vi "I2C Utility Example EEPROM Write-and-Read.vi"() -> ()   [LabVIEW 2020]
panel:
  out "I2C_READ_DATA (Read)":u8[](array[numeric]) format="%x"
  out "Acks Received (Read)":dbl
  in  "I2C_NUM_BYTES_RX (Read)":i32=15
  in  "I2C_WRITE_DATA (Read)":i32[](array[numeric])=[0]
  out "I2C COM Error Out":errorcluster={"status"=FALSE, "code"=0, "source"="No Error"}
  in  "I2C_NUM_BYTES_RX (Write)":i32
  in  "I2C_WRITE_DATA (Write)":u8[](array[numeric])=[0, 222, 173, 190, 239, 1, 2, 3, 4, 5, 6, 7, 222, 173, 190, 239] format="%x"
  out "I2C_READ_DATA (Write)":u8[](array[numeric]) format="%x"
  out "Acks Received (Write)":dbl
  in  "I2C_SLAVE_ADDRESS":i32=80
  in  "I2C_OPTIONS":i32
  in  "I2C_SPEED_THROTTLE":i32
  in  "I2C_SCL_DIONUM":i32=1
  in  "I2C_SDA_DIONUM":i32
  out "Error String":string="No Error"
  out "error out":errorcluster
  out "ConnectionType Out":i32
  out "DeviceType Out":i32
  in  "Identifier":string="LJM_idANY"
  in  "ConnectionType":string="LJM_ctANY"
  in  "DeviceType":string="LJM_dtANY"
  # "Before running this program:\n1. Attach a LJTick-DAC to FIO0 and FIO1\n2. Configure Device Opening Settings (DeviceType, ConnectionType, and Identifier)\n3. Configure I2C Settings (I2C_SDA_DIONUM, I2C_SCL_DIONUM, I2C_SPEED_THROTTLE, I2C_OPTIONS, I2C_SLAVE_ADDRESS)\n4. Run the .vi by either 'ctrl+r' or by pressing the \"Run\" button.\n\nThis program combines the two VI's:\n\"I2C Utility Example EEPROM Write.vi\"\n\"I2C Utility Example EEPROM Read.vi\""
  # "Device Opening Settings"
  # "Data [0]"
  # "PageNum"
  # "Data [0]"
  # "PageNum"
  # "Data [0]"
  # "Data [1]"
  # "Data [1]"
  # "Data [2]"
  # "Data [2]"
  # "Data [1]"
  # "Data [3]"
  # "Data [2]"
  # "Data [3]"
  # "..."
  # "Data [3]"
  # "..."
  # "..."
  # "I2C Settings"
  # "Configures the FIO channel that the \nSDA signal should appear on."
  # "Configures the FIO channel that the \nSDA signal should appear on."
  # "Configures the I2C Clock Speed\n (frequency)"
  # "Configures the I2C options"
  # "..."
  # "..."
  # "Data [14]"
  # "Data [14]"
  # "..."
  # "Configure the slave address to be sent \nat the start of each data transfer"
  # "Data [14]"
  # "Errors:"
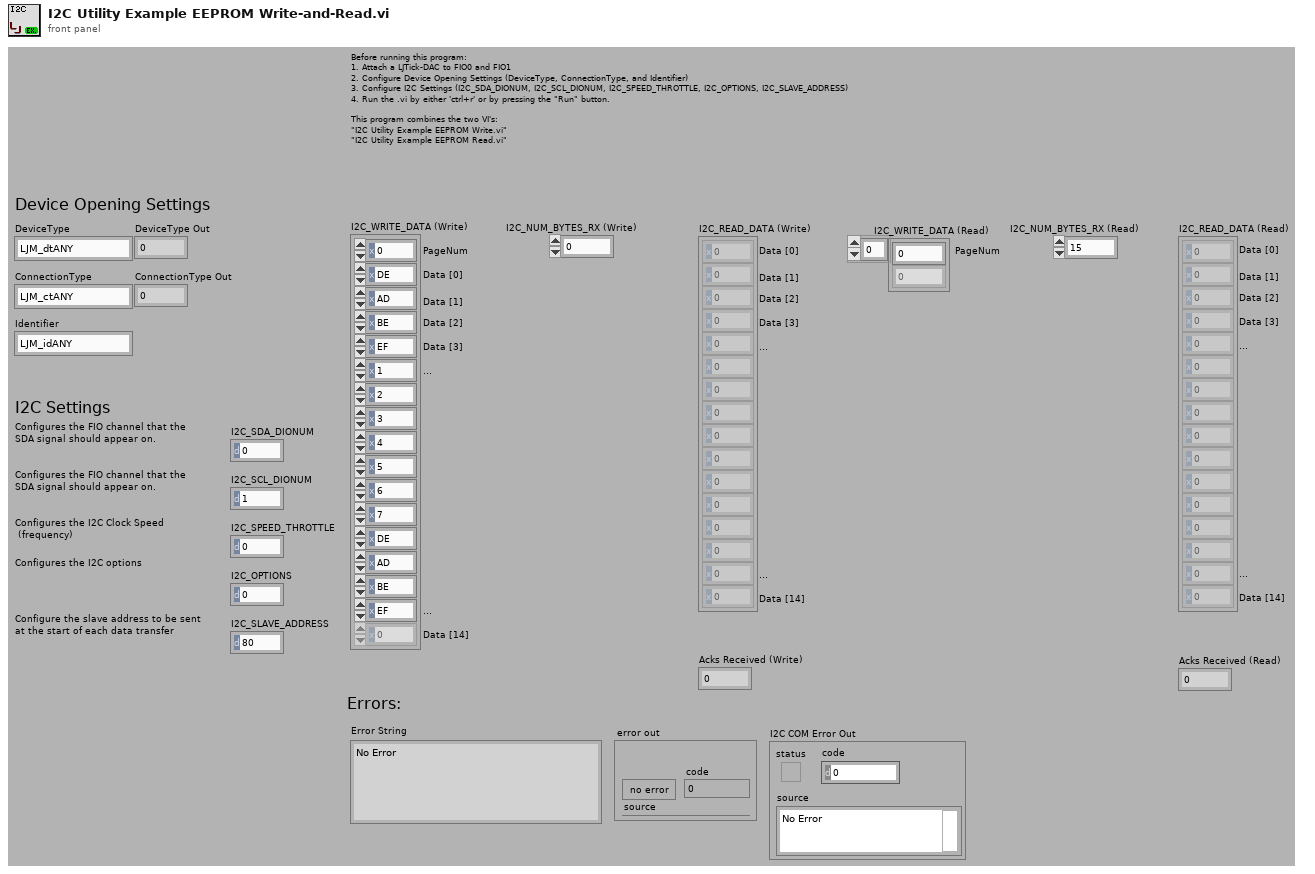
[diagram p1: front panel]
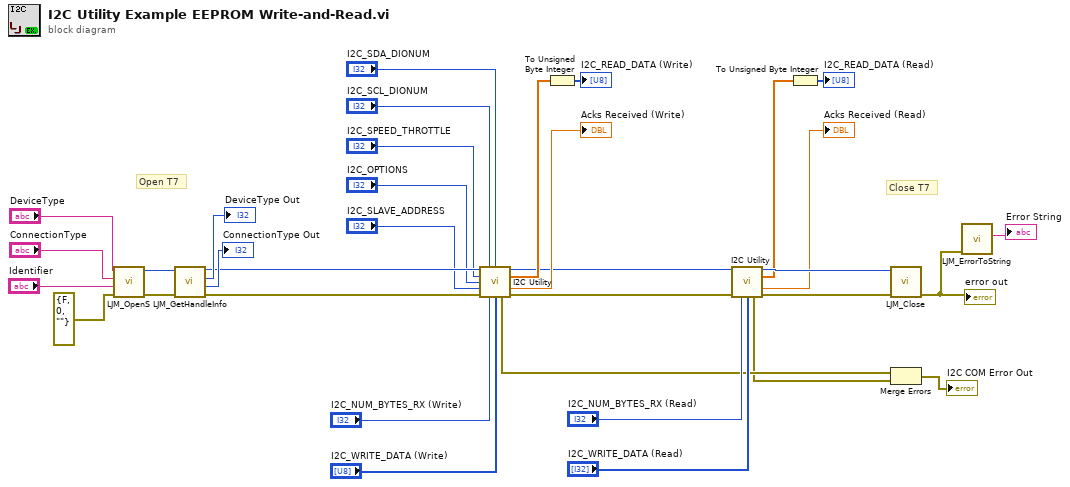
[diagram p0: block diagram]
diagram:
  # "Close T7"
  # "Open T7"
  n1 = call "LJM_OpenS.vi"("error in"=errorcluster {"status"=FALSE, "code"=0, "source"=""} ("error in (no error)"), "Identifier"="Identifier", "ConnectionType"="ConnectionType", "DeviceType"="DeviceType") -> ("error out"=w33:errorcluster, "Handle"=w32:i32)  [unwired: 6 in]
  n2 = call "LJM_GetHandleInfo.vi"("error in"=w33, "Handle In"=w32) -> ("error out"=w23:errorcluster, "ConnectionType"=→"ConnectionType Out":i32, "DeviceType"=→"DeviceType Out":i32, "Handle Out"=w24:i32)  [unwired: 2 in, 4 out]
  n3 = call "I2C Utility.vi"("Handle In"=w24, "I2C_SDA_DIONUM"="I2C_SCL_DIONUM", "I2C_SCL_DIONUM"="I2C_SDA_DIONUM", "I2C_SPEED_THROTTLE"="I2C_SPEED_THROTTLE", "I2C_OPTIONS"="I2C_OPTIONS", "I2C_SLAVE_ADDRESS"="I2C_SLAVE_ADDRESS", "error in"=w23, "I2C_NUM_BYTES_RX"="I2C_NUM_BYTES_RX (Write)", "I2C_WRITE_DATA"="I2C_WRITE_DATA (Write)") -> ("Handle Out"=w10:i32, "Data Read"=w17:dbl[], "Acks Received"=→"Acks Received (Write)":dbl, "I2C COM Error Out"=w2:errorcluster, "error out"=w11:errorcluster)  [unwired: 2 in]
  n4 = To Unsigned Byte Integer(number=w17) -> (unsigned 8bit integer=→"I2C_READ_DATA (Write)":u8[])
  n5 = call "I2C Utility.vi"("Handle In"=w10, "error in"=w11, "I2C_NUM_BYTES_RX"="I2C_NUM_BYTES_RX (Read)", "I2C_WRITE_DATA"="I2C_WRITE_DATA (Read)") -> ("Handle Out"=w9:i32, "Data Read"=w4:dbl[], "Acks Received"=→"Acks Received (Read)":dbl, "I2C COM Error Out"=w1:errorcluster, "error out"=w12:errorcluster)  [unwired: 7 in]
  n6 = To Unsigned Byte Integer(number=w4) -> (unsigned 8bit integer=→"I2C_READ_DATA (Read)":u8[])
  n7 = call "LJM_Close.vi"("error in"=w12, "Handle"=w9) -> ("error out"=w26:errorcluster)  [unwired: 9 in]
  "error out" <- w26
  n8 = Merge Errors(w2, w1) -> (→"I2C COM Error Out":errorcluster)
  n9 = call "LJM_ErrorToString.vi"("error in"=w26) -> ("String"=→"Error String":string)  [unwired: 10 in]
